vi "Example.vi"() -> ()   [LabVIEW 2015]
uses:
  <vilib>/MakerHub/LINX/LMH-LINX.lvlib
panel:
  out "data":T1
  out "Relative Humidity":dbl(slide) scale=0.0..100.0
  out "Temperature":dbl(slide) scale=0.0..50.0
  in  "VISA resource name":refnum<visa-resource-name>="ArduinoUno"
  in  "Delay Time (us)":dbl=3.0 caption="Delay Time (s)"
  in  "Address (0)":i8 format="%x"
  in  "stop":bool
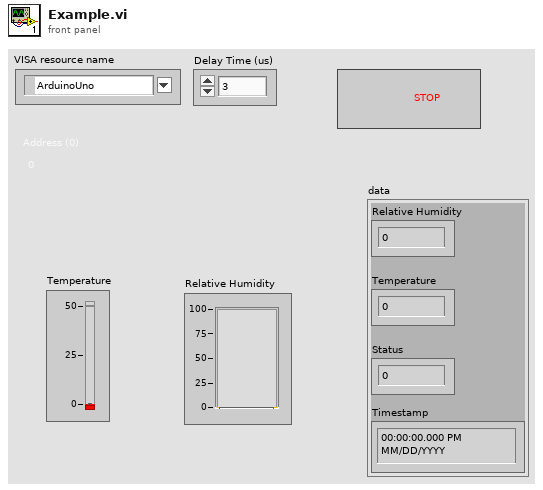
[diagram p1: front panel]
types:
  T1 = cluster{"Relative Humidity":dbl, "Temperature":dbl, "Status":i32, "Timestamp":timestamp}
  T2 = typedef "LMH-LINX.lvlib/LINX Ref.ctl" = cluster{"IO":T3, "Interface":T4, "LINX Device Config":T5}
  T3 = typedef "LMH-LINX.lvlib/Platform.ctl" = enum16{"Remote", "Local"}
  T4 = typedef "LMH-LINX.lvlib/Interface.ctl" = enum16{"Serial", "TCP"}
  T5 = typedef "LMH-LINX.lvlib/Device.lvlib/LINX Device Config.ctl" = cluster{"Interface":T4, "COM Port":refnum<visa-resource-name>, "TCP Configuration":T6, "Device Family":u8, "Device ID":u8, "Device Name":string, "TCP Ref":refnum<k5>, "Channels":T7}
  T6 = typedef "LMH-LINX.lvlib/Device.lvlib/TCP Config.ctl" = cluster{"IP Address":string, "Port":u16}
  T7 = typedef "LMH-LINX.lvlib/Channels.ctl" = cluster{"DI":u8[], "DO":u8[], "AI":u8[], "AO":u8[], "PWM":u8[], "QE":u8[], "UART":u8[], "I2C 2":u8[], "SPI":u8[], "CAN":u8[], "Servo":u8[], "AI Ref (V)":dbl, "AI Resolution (Bits)":u8, "AO Ref (V)":dbl, "AO Resolution (Bits)":u8}
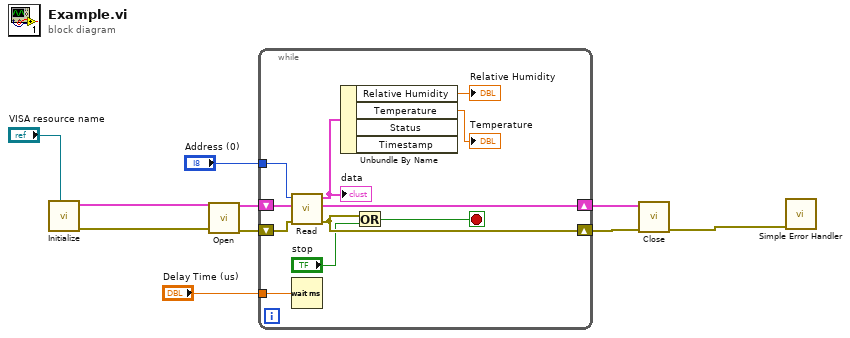
[diagram p0: block diagram]
diagram:
  n1 = call <vilib>:"Initialize.vi"("Serial Port"="VISA resource name") -> ("Error Out"=w9:errorcluster, "LINX Resource"=w6:T2)  [unwired: 8 in, 1 out]
  n2 = call "Open.vi"("error in (no error)"=w9, "LINX Resource in"=w6) -> ("error out"=w8:errorcluster, "LINX Resource out"=w7:T2)  [unwired: 8 in]
  n3 = while {
    shift-right: [w11] -> w3
    shift-left: w7 -> [w20]
    shift-right: [w18] -> w4
    shift-left: w8 -> [w19]
    tunnel: "Address (0)" -> [w21]
    tunnel: "Delay Time (us)" -> [w15]
    stop <- w16 stop-if-true
    n4 = call "Read.vi"("error in (no error)"=w19, "LINX Resource in"=w20, "Address (0x27)"=w21) -> ("error out"=w18:errorcluster, "LINX Resource out"=w11:T2, "data"=w12:T1)  [unwired: 6 in]
    "data" <- w12
    n5 = Wait (ms)(milliseconds to wait=w15) -> ()  [unwired: 1 out]
    n6 = Unbundle By Name(w12) -> ("Relative Humidity"=→"Relative Humidity":dbl, "Temperature"=→"Temperature":dbl)  [unwired: 2 out]
    n7 = Or(x=w18, y="stop") -> (x .or. y?=w16:bool)
  }
  n8 = call <vilib>:"Close.vi"("Error In"=w4, "LINX Resource"=w3) -> ("Error Out"=w5:errorcluster)  [unwired: 9 in]
  n9 = call <vilib>:"Simple Error Handler.vi"("error in (no error)"=w5) -> ()  [unwired: 4 in, 5 out]
